vi "Example Callback.vi"() -> ()   [LabVIEW 2013]
uses:
  C:/tf/play/labview/Tinkerforge.dll
  Tinkerforge.dll
panel:
  out "y":sgl format="%#_13g"
  out "x":sgl format="%#_13g"
  out "w":sgl format="%#_13g"
  in  "stop":bool
  out "z":sgl format="%#_13g"
  in  "uid":string="Ron"
  in  "port":i32=4223
  in  "host":string="localhost"
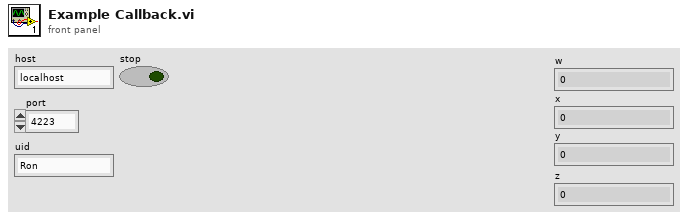
[diagram p1: front panel]
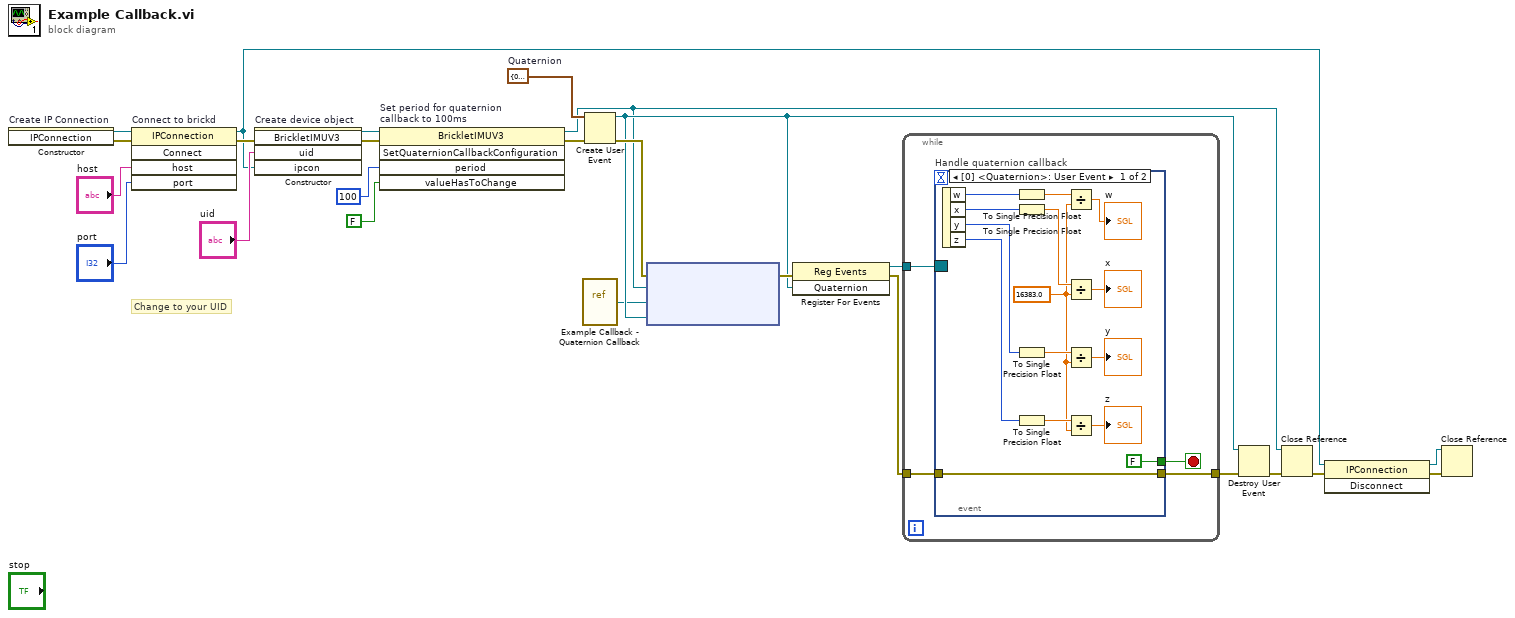
[diagram p0: block diagram]
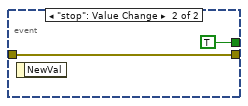
[diagram p2: hidden frame]
diagram:
  w9 = cluster{"w":i16, "x":i16, "y":i16, "z":i16} {"w"=0, "x"=0, "y"=0, "z"=0}  # Quaternion
  # "Change to your UID"
  n1 = constructor on="Create IP Connection" class="IPConnection"() -> (reference out=w25:refnum<k24>, error out=w3:errorcluster)  [unwired: 3 in, 1 out]
  n2 = invoke on="Connect to brickd" class="IPConnection" method="Connect"(reference=w25, error in=w3, "host"="host", "port"="port") -> (reference out=w18:refnum<k24>, error out=w21:errorcluster)  [unwired: 1 in, 3 out]
  n3 = constructor on="Create device object" class="BrickletIMUV3"(error in=w21, "uid"="uid", "ipcon"=w18) -> (reference out=w6:refnum<k24>, error out=w8:errorcluster)  [unwired: 2 in, 3 out]
  n4 = invoke on="Set period for quaternion\ncallback to 100ms" class="BrickletIMUV3" method="SetQuaternionCallbackConfiguration"(reference=w6, error in=w8, "period"=i64 100, "valueHasToChange"=FALSE) -> (reference out=w5:refnum<k24>, error out=w7:errorcluster)  [unwired: 1 in, 3 out]
  n5 = vi-ref "Example Callback - Quaternion Callback.vi"() -> ("vi reference"=w1:refnum<vi>)
  n6 = Create User Event(user event datatype=w9, error in=w7) -> (user event=w11:refnum<user-event>, error out=w16:errorcluster)
  n7 = node ("Register Event Callback")(w16, w5, w1, w11) -> (w15:errorcluster)  [unwired: 1 in, 1 out]
  n8 = register-events(error in=w15, w11) -> (reference out=w14:refnum<event-registration>, error out=w12:errorcluster)  [unwired: 1 in]
  n9 = while {
    tunnel: w14 -> [w29]
    tunnel: [w28] -> w13
    tunnel: w12 -> [w27]
    stop <- w26 stop-if-true
    n10 = event "Handle quaternion callback" shown="[0] <Quaternion>: User Event" {
      selector: w29 -> [_ _]
      dyn-events: _ -> [_ _]
      timeout: _ -> [_ _]
      tunnel: [w44 w45] -> w28
      tunnel: w27 -> [w44 w45]
      tunnel: [FALSE TRUE] -> w26
      event User Event {
        w30 = sgl 16383.0 ("y")
        n11 = event-data() -> ("w"=w41:i16, "x"=w33:i16, "y"=w32:i16, "z"=w31:i16)  [unwired: 1 in]
        n12 = To Single Precision Float(number=w41) -> (single precision float=w40:sgl)
        n13 = To Single Precision Float(number=w33) -> (single precision float=w39:sgl)
        n14 = To Single Precision Float(number=w32) -> (single precision float=w38:sgl)
        n15 = To Single Precision Float(number=w31) -> (single precision float=w37:sgl)
        n16 = Divide(x=w40, y=w30) -> (x/y=→"w":sgl)
        n17 = Divide(x=w39, y=w30) -> (x/y=→"x":sgl)
        n18 = Divide(x=w38, y=w30) -> (x/y=→"y":sgl)
        n19 = Divide(x=w37, y=w30) -> (x/y=→"z":sgl)
      }
      event "stop": Value Change {
        n20 = event-data() -> ()  [unwired: 1 in, 1 out]
      }
    }
  }
  n21 = Destroy User Event(user event=w11, error in=w13) -> (error out=w10:errorcluster)
  n22 = Close Reference(reference=w5, error in (no error)=w10) -> (error out=w20:errorcluster)
  n23 = invoke class="IPConnection" method="Disconnect"(reference=w18, error in=w20) -> (reference out=w17:refnum<k24>, error out=w19:errorcluster)  [unwired: 1 in, 1 out]
  n24 = Close Reference(reference=w17, error in (no error)=w19) -> ()  [unwired: 1 out]
